vi "Edit List.vi"(6 "Selected Line":i32, 7 "Method":T1(ring), 8 "error in (no error)":errorcluster, 9 "Alias":string, 10 "IP Address":string, 11 "IP List":refnum<vi>) -> (0 "error out":errorcluster, 1 "Alias":string, 2 "IP Address":string, 4 "Selected Line":i32)   [LabVIEW 2014]
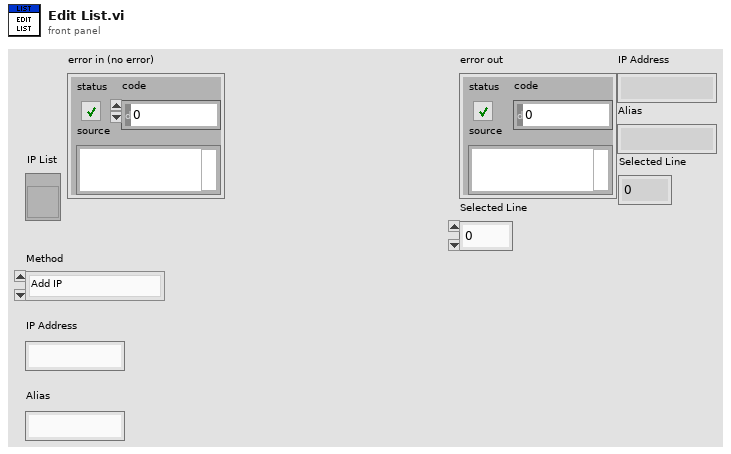
[diagram p1: front panel]
types:
  T1 = enum16{"Add IP", "Delete IP", "Get IP", "Edit IP"}
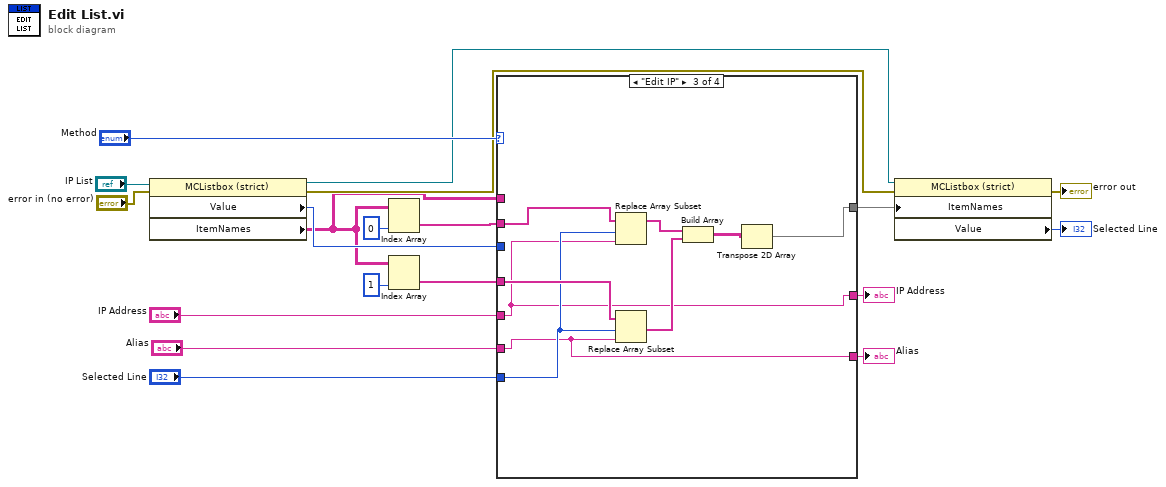
[diagram p0: block diagram]
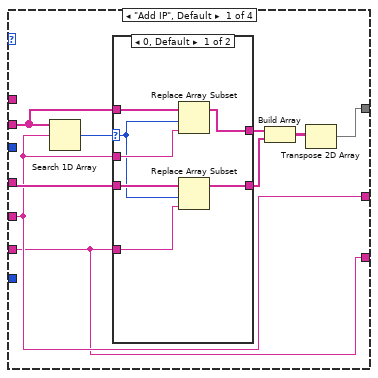
[diagram p2: hidden frame]
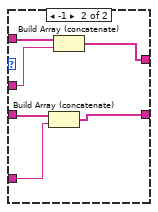
[diagram p3: hidden frame]
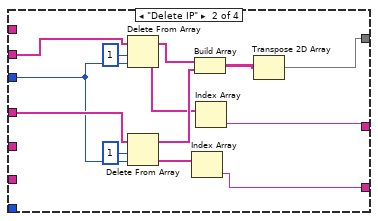
[diagram p4: hidden frame]
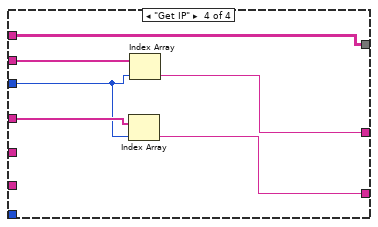
[diagram p5: hidden frame]
diagram:
  n1 = property class="MCListbox (strict)"(reference="IP List", error in="error in (no error)") -> (reference out=w8:refnum<vi>, error out=w7:errorcluster, "Value"=w6:i32, "ItemNames"=w5:string[][])
  n2 = Index Array(array=w5, index (col)=0 ("disabled index (col)")) -> (element=w12:string[])  [unwired: 1 in]
  n3 = Index Array(array=w5, index (col)=1 ("disabled index (col)")) -> (element=w11:string[])  [unwired: 1 in]
  n4 = case shown="\"Edit IP\"" "Method" {
    tunnel: w12 -> [w27 w53 w63 w68]
    tunnel: "IP Address" -> [w21 _ w56 _]
    tunnel: w11 -> [w26 w52 w62 w67]
    tunnel: [w22 w47 w60 w69] -> w10
    tunnel: "Alias" -> [w20 _ w55 _]
    tunnel: w6 -> [_ w46 _ w66]
    tunnel: w5 -> [_ _ _ w69]
    tunnel: [w21 w43 w56 w65] -> w4
    tunnel: [w20 w44 w55 w64] -> w3
    tunnel: "Selected Line" -> [_ _ w59 _]
    frame "Add IP", Default {
      n5 = Search 1D Array(1D array=w27, element=w21) -> (index of element=w28:i32)  [unwired: 1 in]
      n6 = case shown="0, Default" w28 {
        selector: w28 -> [w31 _]
        tunnel: w27 -> [w35 w41]
        tunnel: w21 -> [w32 w40]
        tunnel: w26 -> [w34 w39]
        tunnel: w20 -> [w33 w38]
        tunnel: [w30 w36] -> w24
        tunnel: [w29 w37] -> w23
        frame 0, Default {
          n7 = Replace Array Subset(array=w35, new element=w32, index=w31) -> (w30:string[])
          n8 = Replace Array Subset(array=w34, new element=w33, index=w31) -> (w29:string[])
        }
        frame -1 {
          n9 = Build Array (concatenate)(w39, w38) -> (w37:string[])
          n10 = Build Array (concatenate)(w41, w40) -> (w36:string[])
        }
      }
      n11 = Build Array(w24, w23) -> (w25:string[][])
      n12 = Transpose 2D Array(2D array=w25) -> (transposed array=w22:string[][])
    }
    frame "Delete IP" {
      n13 = Delete From Array(array=w53, length=1, index=w46) -> (deleted portion=w42:string[], array with subset deleted=w49:string[])
      n14 = Delete From Array(array=w52, length=1, index=w46) -> (deleted portion=w45:string[], array with subset deleted=w50:string[])
      n15 = Index Array(array=w45) -> (element=w44:string)  [unwired: 1 in]
      n16 = Build Array(w49, w50) -> (w48:string[][])
      n17 = Index Array(array=w42) -> (element=w43:string)  [unwired: 1 in]
      n18 = Transpose 2D Array(2D array=w48) -> (transposed array=w47:string[][])
    }
    frame "Edit IP" {
      n19 = Replace Array Subset(array=w63, new element=w56, index=w59) -> (w58:string[])
      n20 = Replace Array Subset(array=w62, new element=w55, index=w59) -> (w57:string[])
      n21 = Build Array(w58, w57) -> (w61:string[][])
      n22 = Transpose 2D Array(2D array=w61) -> (transposed array=w60:string[][])
    }
    frame "Get IP" {
      n23 = Index Array(array=w67, index=w66) -> (element=w64:string)
      n24 = Index Array(array=w68, index=w66) -> (element=w65:string)
    }
  }
  "IP Address" <- w4
  "Alias" <- w3
  n25 = property class="MCListbox (strict)"(reference=w8, error in=w7, "ItemNames"=w10) -> (error out=→"error out":errorcluster, "Value"=→"Selected Line":i32)  [unwired: 1 out]
